vi "Digital_Input_8Channels.vi"(1 "IO":T1={"DI 0"="Mod1/DIO2", "DI 1"="Mod1/DIO2", "DI 2"="Mod1/DIO2", "DI 3"="Mod1/DIO2", "DI 4"="Mod1/DIO2", "DI 5"="Mod1/DIO2", "DI 6"="Mod1/DIO2", "DI 7"="Mod1/DIO2"}) -> (0 "States":bool[](array[boolean]))   [LabVIEW 2015]
uses:
  <vilib>/rvi/eio/common/nirviEmuTemplateMethod_errors.vi
  <vilib>/eio/EIONode/EIONode.xnode
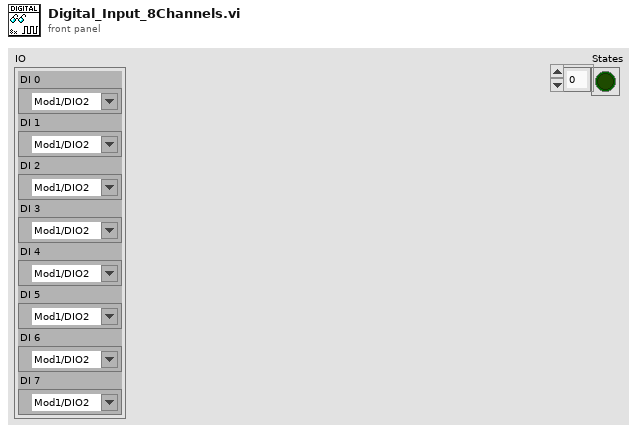
[diagram p1: front panel]
types:
  T1 = cluster{"DI 0":refnum<k21>, "DI 1":refnum<k21>, "DI 2":refnum<k21>, "DI 3":refnum<k21>, "DI 4":refnum<k21>, "DI 5":refnum<k21>, "DI 6":refnum<k21>, "DI 7":refnum<k21>}
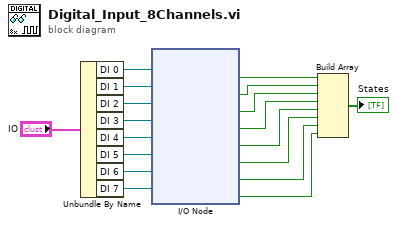
[diagram p0: block diagram]
diagram:
  n1 = Unbundle By Name("IO") -> ("DI 0"=w17:refnum<k21>, "DI 1"=w16:refnum<k21>, "DI 2"=w15:refnum<k21>, "DI 3"=w14:refnum<k21>, "DI 4"=w13:refnum<k21>, "DI 5"=w12:refnum<k21>, "DI 6"=w11:refnum<k21>, "DI 7"=w10:refnum<k21>)
  n2 = xnode "I/O Node"("FPGA I/O In"=w17, "FPGA I/O In"=w16, "FPGA I/O In"=w15, "FPGA I/O In"=w14, "FPGA I/O In"=w13, "FPGA I/O In"=w12, "FPGA I/O In"=w11, "FPGA I/O In"=w10) -> ("I/O Item"=w9:bool, "I/O Item"=w8:bool, "I/O Item"=w7:bool, "I/O Item"=w6:bool, "I/O Item"=w5:bool, "I/O Item"=w4:bool, "I/O Item"=w3:bool, "I/O Item"=w2:bool)  [unwired: 8 out]
  n3 = Build Array(w9, w8, w7, w6, w5, w4, w3, w2) -> (→"States":bool[])
